vi "svx_DAQ_ControlSizes.vi"() -> (3 "Task Configuration Pane Heights":u32[](array[numeric])=[269, 225, 181], 4 "XControl Sizes":T1[](array[typedef])=[{"Width"=601, "Height"=289}, {"Width"=601, "Height"=245}, {"Width"=601, "Height"=201}], 6 "Buttons Top - Pixel Values":i32[](array[numeric])=[269, 225, 181], 8 "Error Image Top - Pixel Values":i32[](array[numeric])=[263, 219, 175], 10 "Enable Logging Top - Pixel Values":i32[](array[numeric])=[263, 219, 175], 15 "Logfile Path Top - Pixel Values":i32[](array[numeric])=[263, 219, 175])   [LabVIEW 2017, in "SVX NI-DAQmx AI Configuration XControl.xctl"]
uses:
  <vilib>/addons/Sound and Vibration/svt_DAQmx/Configuration XControl/SVX NI-DAQmx AI Configuration XControl.xctl
  <vilib>/Utility/miscctls.llb/LVBoundsTypeDef.ctl
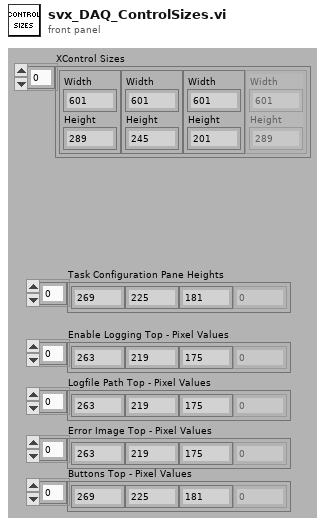
[diagram p1: front panel]
types:
  T1 = typedef "LVBoundsTypeDef.ctl" = cluster{"Width":u32, "Height":u32}
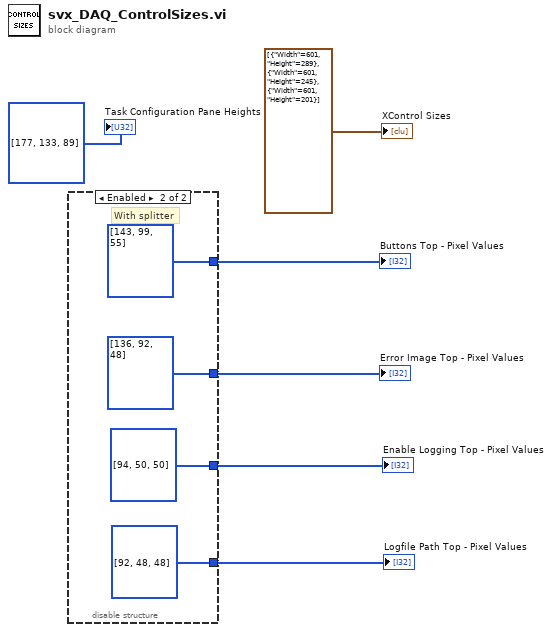
[diagram p0: block diagram]
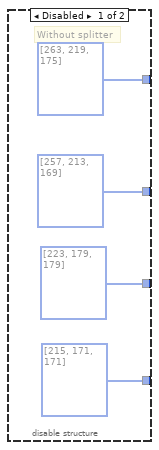
[diagram p2: hidden frame]
diagram:
  n1 = disable-structure shown="Enabled" {
    disable-tunnel: [i32[] [263, 219, 175] i32[] [143, 99, 55]] -> w4
    disable-tunnel: [i32[] [257, 213, 169] i32[] [136, 92, 48]] -> w3
    disable-tunnel: [i32[] [223, 179, 179] i32[] [94, 50, 50]] -> w2
    disable-tunnel: [i32[] [215, 171, 171] i32[] [92, 48, 48]] -> w1
    frame Disabled {
      # "Without splitter"
    }
    frame Enabled {
      # "With splitter"
    }
  }
  "Buttons Top - Pixel Values" <- w4
  "Error Image Top - Pixel Values" <- w3
  "Enable Logging Top - Pixel Values" <- w2
  "Logfile Path Top - Pixel Values" <- w1
  "XControl Sizes" <- T1[] [{"Width"=601, "Height"=289}, {"Width"=601, "Height"=245}, {"Width"=601, "Height"=201}]
  "Task Configuration Pane Heights" <- u32[] [177, 133, 89] ("Task Configuration Panel Heights")
